vi "pub_bool.vi"() -> ()   [LabVIEW 2019]
uses:
  <vilib>/RTI DDS Toolkit/Types/RTI DDS Advanced Writer Configuration.ctl
  <vilib>/RTI DDS Toolkit/VIs/AdvancedCreateWriter_Bool.vi
  <vilib>/RTI DDS Toolkit/VIs/Write_Bool.vi
  <vilib>/RTI DDS Toolkit/Library/LVDDS_library.lvlib
panel:
  in  "dt":u32=500
  in  "Topic Name":string="rt/lvbool"
  in  "Data":bool
  in  "stop":bool
  in  "Advanced Writer Configuration":T1={"typeName"="std_msgs::msg::dds_::Bool_", "keyName"="", "domainParticipantQoSProfile"="", "dataWriterQoSProfile"="", "forceArrayMapping?"=FALSE, "forceUnboundedString?"=FALSE}
  in  "Domain Id":u32
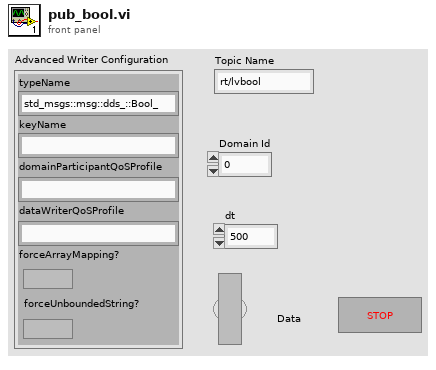
[diagram p1: front panel]
types:
  T1 = typedef "LVDDS_library.lvlib/RTI DDS Advanced Writer Configuration.ctl" = cluster{"typeName":string, "keyName":string, "domainParticipantQoSProfile":string, "dataWriterQoSProfile":string, "forceArrayMapping?":bool, "forceUnboundedString?":bool}
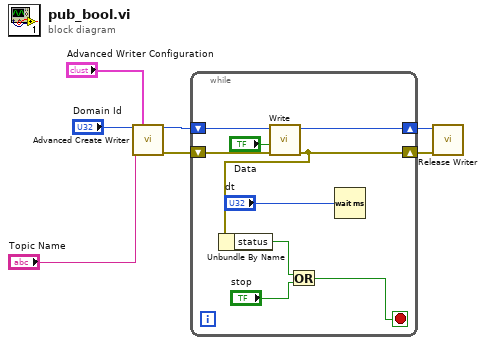
[diagram p0: block diagram]
diagram:
  n1 = call-poly <vilib>:"Advanced Create Writer.vi"("Domain Id"="Domain Id", "Advanced Writer Configuration"="Advanced Writer Configuration", "Topic Name"="Topic Name") -> ("DDS Object Ref"=w7:u64, "error out"=w4:errorcluster)  [unwired: 11 in]
  n2 = while {
    shift-right: [w15] -> w6
    shift-left: w7 -> [w16]
    shift-right: [w13] -> w5
    shift-left: w4 -> [w14]
    stop <- w11 stop-if-true
    n3 = call-poly <vilib>:"Write.vi"("error in (no error)"=w14, "Data"="Data", "DDS Object Ref in"=w16) -> ("error out"=w13:errorcluster, "DDS Object Ref out"=w15:u64)  [unwired: 7 in]
    n4 = Unbundle By Name(w13) -> ("status"=w12:bool)
    n5 = Or(x=w12, y="stop") -> (x .or. y?=w11:bool)
    n6 = Wait (ms)(milliseconds to wait="dt") -> ()  [unwired: 1 out]
  }
  n7 = call <vilib>:"Release Writer.vi"("error in (no error)"=w5, "DDS Object Ref"=w6) -> ()  [unwired: 9 in, 1 out]
